vi "Trigger subv frames based.vi"(0 "T=continuous, F=finite":bool, 2 "Initial delay\n[frames]":dbl=2.0 min=0.1 step=1.0, 3 "Pulse duration [ms]":dbl=2.0 min=0.1 step=1.0, 4 "Pulse\nevery n frames":i32=2 min=1 max=10000 step=1, 5 "Sample clock rate":dbl, 6 "ADsamples.per.frame":dbl=20000.0 format="%#_6e", 7 "pixel.dwell.time.in.ticks":dbl=20000.0, 9 "pixel.dwell.time.in.sec":dbl=2.0 min=0.1 step=1.0) -> (14 "ctr tasks out":refnum<k21>[](array[refnum]), 19 "error out":errorcluster)   [LabVIEW 2012]
doc: "SciScan 1.2 160622"
uses:
  <vilib>/DAQmx/create/channels.llb/DAQmx Create Channel (CO-Pulse Generation-Ticks).vi
  <vilib>/DAQmx/configure/timing.llb/DAQmx Timing (Implicit).vi
panel:
  # "1.31072E+6"
  # "20"
  # "4E-6"
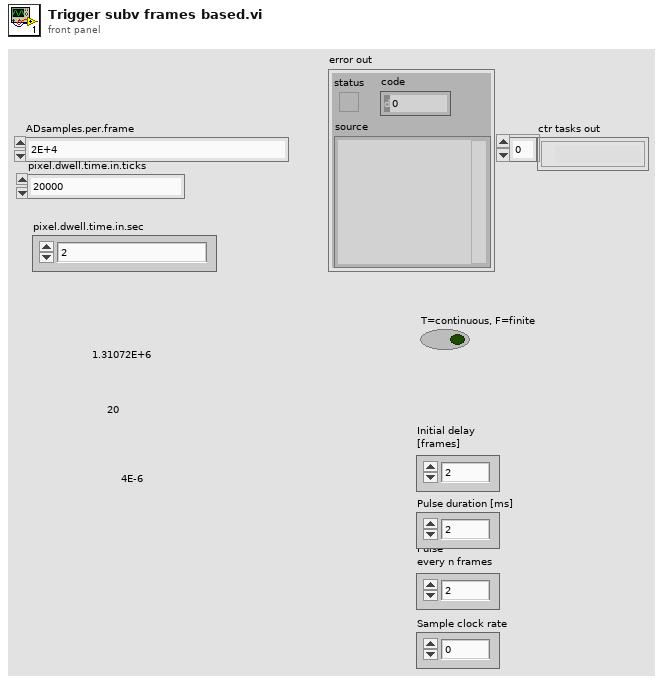
[diagram p1: front panel]
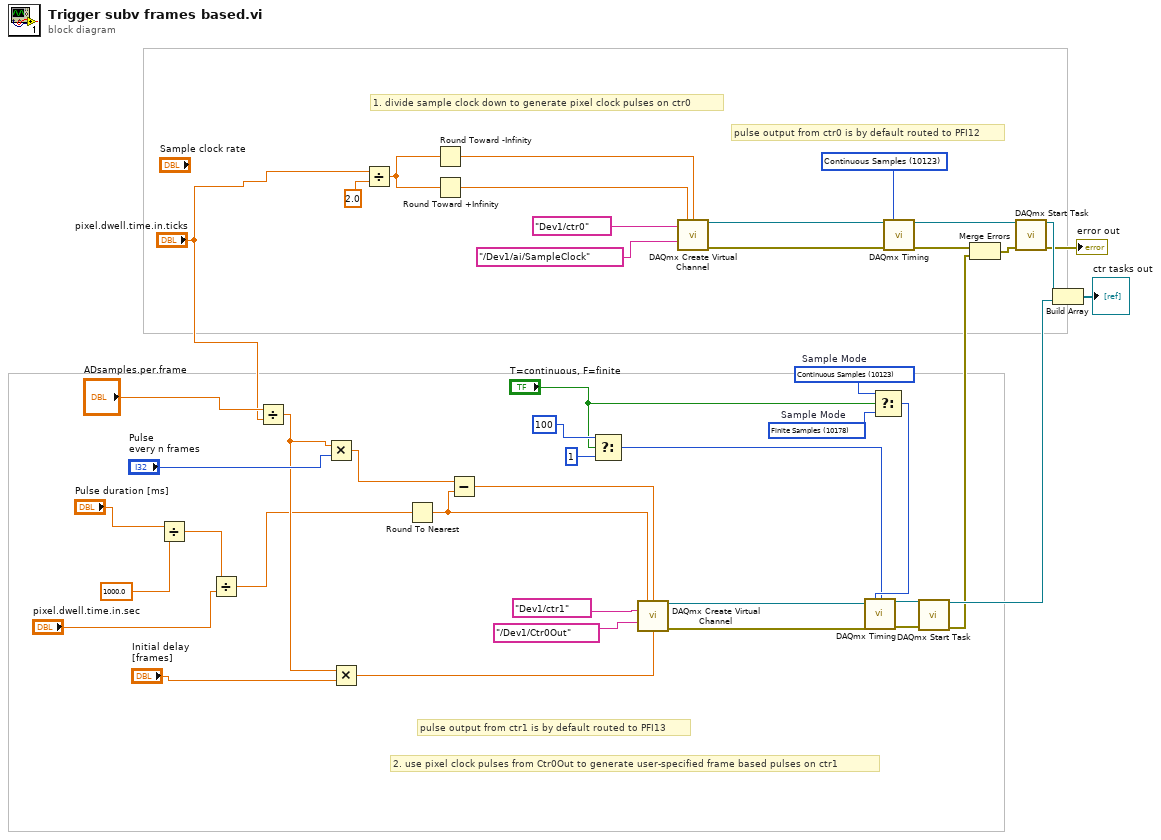
[diagram p0: block diagram]
diagram:
  w19 = 10123 items=["Finite Samples"=10178, "Continuous Samples"=10123, "Hardware Timed Single Point"=12522] ("sample mode")
  w38 = 10123 items=["Finite Samples"=10178, "Continuous Samples"=10123, "Hardware Timed Single Point"=12522]  # Sample Mode
  w39 = 10178 items=["Finite Samples"=10178, "Continuous Samples"=10123, "Hardware Timed Single Point"=12522]  # Sample Mode
  # "pulse output from ctr1 is by default routed to PFI13"
  # "pulse output from ctr0 is by default routed to PFI12"
  # "2. use pixel clock pulses from Ctr0Out to generate user-specified frame based pulses on ctr1"
  # "1. divide sample clock down to generate pixel clock pulses on ctr0"
  n1 = Divide(x="Pulse duration [ms]", y=1000.0) -> (x/y=w8:dbl)
  n2 = Divide(x=w8, y="pixel.dwell.time.in.sec") -> (x/y=w6:dbl)
  n3 = Divide(x="ADsamples.per.frame", y="pixel.dwell.time.in.ticks") -> (x/y=w14:dbl)
  n4 = Multiply(x=w14, y="Pulse\nevery n frames") -> (x*y=w15:dbl)
  n5 = Multiply(x=w14, y="Initial delay\n[frames]") -> (x*y=w42:dbl)
  n6 = Divide(x="pixel.dwell.time.in.ticks", y=2.0 ("x")) -> (x/y=w12:dbl)
  n7 = Round To Nearest(number=w6) -> (nearest integer value=w5:dbl)
  n8 = Round Toward -Infinity(1:w12) -> (0:w28:dbl)
  n9 = Round Toward +Infinity(x=w12) -> (ceil(x): smallest int >= x=w29:dbl)
  n10 = Subtract(x=w15, y=w5) -> (x-y=w13:dbl)
  n11 = Select(t=100, s="T=continuous, F=finite", f=1) -> (s? t:f=w36:i32)
  n12 = call-poly <vilib>:"DAQmx Create Virtual Channel.vi"("high ticks"=w5, "low ticks"=w13, "counter"=tag "Dev1/ctr1", "source of ticks"=tag "/Dev1/Ctr0Out", "initial delay"=w42) -> ("task out"=w1:refnum<k21>, "error out"=w2:errorcluster)  [unwired: 9 in]
  n13 = call-poly <vilib>:"DAQmx Create Virtual Channel.vi"("high ticks"=w29, "low ticks"=w28, "counter"=tag "Dev1/ctr0", "source of ticks"=tag "/Dev1/ai/SampleClock") -> ("task out"=w31:refnum<k21>, "error out"=w32:errorcluster)  [unwired: 10 in]
  n14 = Select(t=w38, s="T=continuous, F=finite", f=w39) -> (s? t:f=w37:i32)
  n15 = call-poly <vilib>:"DAQmx Timing.vi"("task/channels in"=w1, "sample mode"=w37, "samples per channel"=w36, "error in"=w2) -> ("task out"=w40:refnum<k21>, "error out"=w41:errorcluster)  [unwired: 10 in]
  n16 = call-poly <vilib>:"DAQmx Timing.vi"("task/channels in"=w31, "sample mode"=w19, "error in"=w32) -> ("task out"=w25:refnum<k21>, "error out"=w24:errorcluster)  [unwired: 11 in]
  n17 = call <vilib>:"DAQmx Start Task.vi"("task/channels in"=w40, "error in"=w41) -> ("task out"=w33:refnum<k21>, "error out"=w23:errorcluster)  [unwired: 12 in]
  n18 = Merge Errors(w24, w23) -> (w22:errorcluster)
  n19 = call <vilib>:"DAQmx Start Task.vi"("task/channels in"=w25, "error in"=w22) -> ("task out"=w21:refnum<k21>, "error out"=→"error out":errorcluster)  [unwired: 12 in]
  n20 = Build Array(w21, w33) -> (→"ctr tasks out":refnum<k21>[])
